vi "LH_InitList.vi"(2 "InputContents":i32[](array[numeric]), 3 "InputList":refnum<class "ListHead.lvclass">) -> (1 "OutputList":refnum<class "ListHead.lvclass">)   [LabVIEW 2014, in "ListHead.lvclass"]
uses:
  ListHead.lvclass
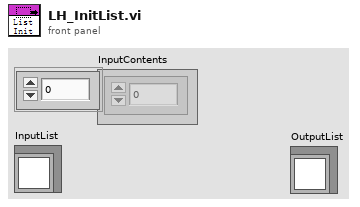
[diagram p1: front panel]
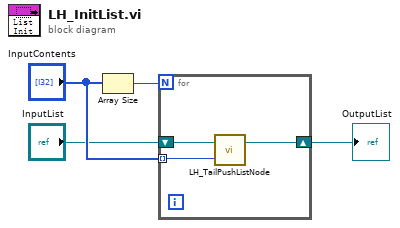
[diagram p0: block diagram]
diagram:
  n1 = Array Size(array="InputContents") -> (size(s)=w4:i32)
  n2 = for {
    N: w4 -> [_]
    tunnel: "InputContents" -> [w6] mode=indexing
    shift-right: [w5] -> w1
    shift-left: "InputList" -> [w7]
    n3 = call "LH_TailPushListNode.vi"("Content"=w6, "InputList"=w7) -> ("OutputList"=w5:refnum<class "ListHead.lvclass">)  [unwired: 1 in]
  }
  "OutputList" <- w1
